vi "LaserStartUpSequence.vi"(8 "error in (no error)":errorcluster) -> (0 "error out":errorcluster)   [LabVIEW 2011]
uses:
  Variables/405Pico.vi
  Variables/625CubeLaser.vi
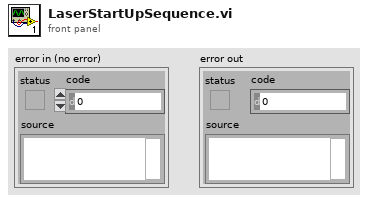
[diagram p1: front panel]
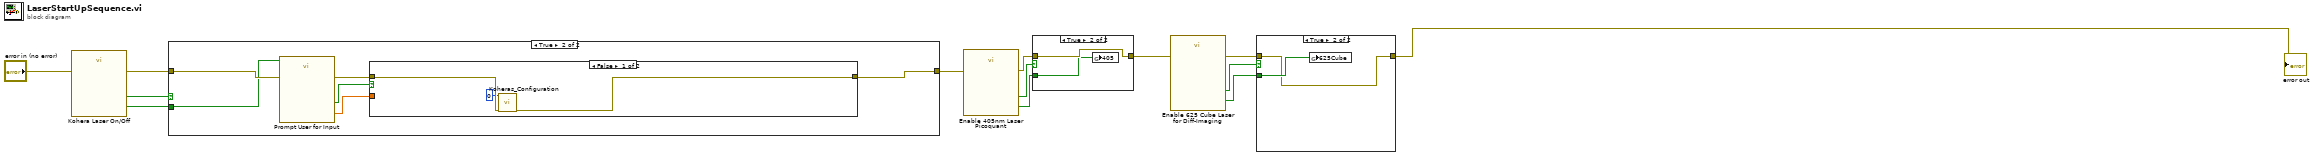
[diagram p0: block diagram]
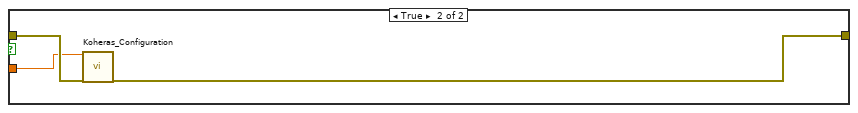
[diagram p3: hidden frame]
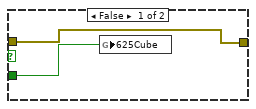
[diagram p4: hidden frame]
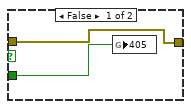
[diagram p5: hidden frame]
diagram:
  n1 = call "Kohera Laser On/Off"("error in (no error)"="error in (no error)") -> ("Koheras Laser On/Off"=w13:bool, "OK"=w12:bool, "error out"=w11:errorcluster)  [unwired: 16 in]
  n2 = case shown="True" w12 {
    tunnel: [w14 w17] -> w1
    tunnel: w11 -> [w14 w16]
    tunnel: w13 -> [_ w15]
    frame False {
    }
    frame True {
      n3 = call "Prompt User for Input"("Enable"=w15, "error in (no error)"=w16) -> ("Laser Power"=w19:dbl, "OK"=w18:bool, "error out"=w20:errorcluster)  [unwired: 15 in]
      n4 = case shown="False" w18 {
        tunnel: [w22 w26] -> w17
        tunnel: w20 -> [w23 w25]
        tunnel: w19 -> [_ w24]
        frame False {
          n5 = call "Koheras_Configuration.vi"("laserPower"=0, "error in"=w23) -> ("out"=w22:errorcluster)  [unwired: 17 in]
        }
        frame True {
          n6 = call "Koheras_Configuration.vi"("laserPower"=w24, "error in"=w25) -> ("out"=w26:errorcluster)  [unwired: 17 in]
        }
      }
    }
  }
  n7 = call "Enable 405nm Laser Picoquant"("error in (no error)"=w1) -> ("On/Off"=w4:bool, "OK"=w3:bool, "error out"=w2:errorcluster)  [unwired: 16 in]
  n8 = case shown="True" w3 {
    tunnel: [w28 w30] -> w8
    tunnel: w2 -> [w28 w30]
    tunnel: w4 -> [w27 w29]
    frame False {
      n9 = global write "405Pico.vi" "405"(w27) -> ()
    }
    frame True {
      n10 = global write "405Pico.vi" "405"(w29) -> ()
    }
  }
  n11 = call "Enable 625 Cube Laser for Diff-Imaging"("error in (no error)"=w8) -> ("On/Off"=w7:bool, "OK"=w6:bool, "error out"=w5:errorcluster)  [unwired: 16 in]
  n12 = case shown="True" w6 {
    tunnel: [w32 w33] -> w9
    tunnel: w5 -> [w32 w33]
    tunnel: w7 -> [w31 w34]
    frame False {
      n13 = global write "625CubeLaser.vi" "625Cube"(w31) -> ()
    }
    frame True {
      n14 = global write "625CubeLaser.vi" "625Cube"(w34) -> ()
    }
  }
  "error out" <- w9
